vi "overlay_spot_circle.vi"(2 "Bubble Size":dbl, 4 "ID":dbl, 5 "error in":errorcluster, 6 "color(black)":u32, 7 "Position":cluster{"x":dbl, "y":dbl, "z":dbl}, 8 "image":T3) -> (0 "error out":errorcluster, 3 "Image Out":T3)   [LabVIEW 2019]
uses:
  <vilib>/vision/Image Controls.llb/IMAQ Image.ctl
  spot.ctl
  line_trapping.ctl
panel:
  in  "Spot Storage":T1[](array[typedef]) {"Amplitude Correction" step=0.1; "Line Trapping"."Phase Gradient" step=0.05; "Line Trapping"."Vector"."x" step=1e-06 format="%#_6p"; "Line Trapping"."Vector"."y" step=1e-06 format="%#_6p"; "Line Trapping"."Vector"."z" step=1e-06 format="%#_6p"; "NA Position"."r" step=1e-06; "NA Position"."y" step=1e-06; "NA Position"."x" step=1e-06; "Position"."z" step=1e-06; "Position"."y" step=1e-06; "Position"."x" step=1e-06; "Phase" step=0.7753; "Intensity" step=0.1}
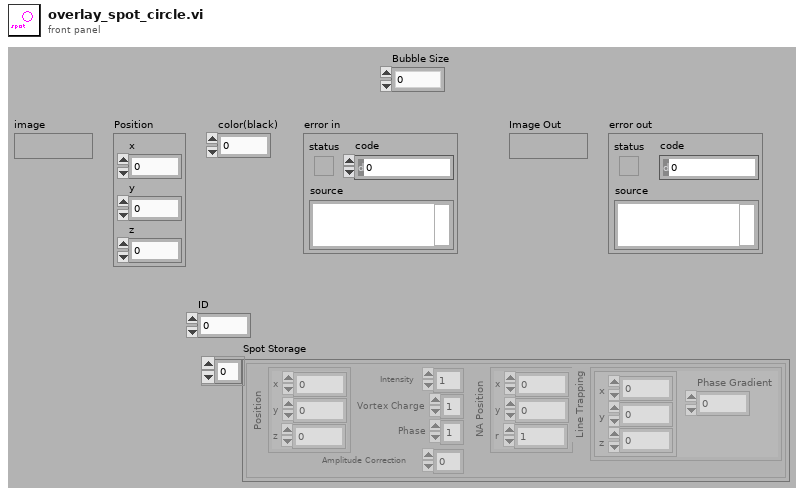
[diagram p1: front panel]
types:
  T1 = typedef "spot.ctl" = cluster{"Position":cluster{"x":dbl, "y":dbl, "z":dbl}, "Intensity":dbl, "Vortex Charge":i8, "Phase":dbl, "NA Position":cluster{"x":dbl, "y":dbl, "r":dbl}, "Line Trapping":T2, "Amplitude Correction":dbl}
  T2 = typedef "line_trapping.ctl" = cluster{"Vector":cluster{"x":dbl, "y":dbl, "z":dbl}, "Phase Gradient":dbl}
  T3 = typedef "IMAQ Image.ctl" = refnum<image>
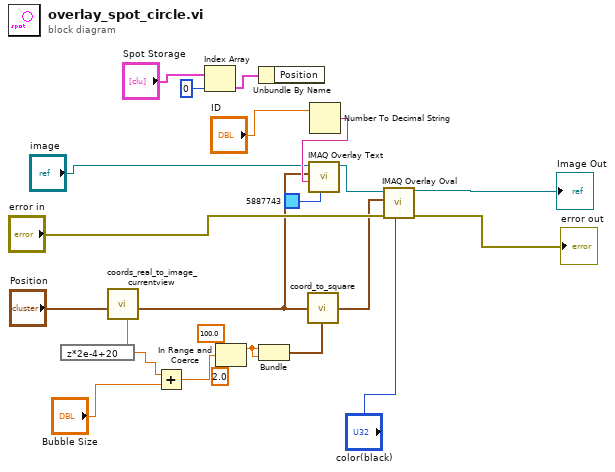
[diagram p0: block diagram]
diagram:
  n1 = call "coords_real_to_image_currentview.vi"("Position (real coords)"="Position") -> ("Position (pixels, relative to the top left of the image)"=w10:cluster{dbl, dbl}, "z (real coords)"=w19:dbl)  [unwired: 7 in]
  n2 = expression code="z*2e-4+20"(w19) -> (w3:dbl)
  n3 = Add(x=w3, y="Bubble Size") -> (x+y=w1:dbl)
  n4 = Index Array(array="Spot Storage", index=0) -> (element=w5:T1)
  n5 = In Range and Coerce(upper limit=100.0, x=w1, lower limit=2.0) -> (coerced(x)=w20:dbl)  [unwired: 1 out]
  n6 = Unbundle By Name(w5) -> ()  [unwired: 1 out]
  n7 = Bundle("upper limit"=w20, "upper limit"=w20) -> (w16:cluster{"upper limit":dbl, "upper limit":dbl})  [unwired: 1 in]
  n8 = call "coord_to_square.vi"("Size"=w16, "Centre"=w10) -> ("rectangle"=w21:cluster{dbl, dbl, dbl, dbl})  [unwired: 2 in]
  n9 = Number To Decimal String(number="ID") -> (decimal integer string=w12:string)  [unwired: 1 in]
  n10 = call "IMAQ Overlay Text"("Text Color (black)"=u32 5887743, "String"=w12, "Origin"=w10, "Image"="image") -> ("Image Out"=w9:T3)  [unwired: 6 in, 1 out]
  n11 = call "IMAQ Overlay Oval"("Color"="color(black)", "error in (no error)"="error in", "Bounding Rectangle"=w21, "Image"=w9) -> ("error out"=→"error out":errorcluster, "Image Out"=→"Image Out":T3)  [unwired: 6 in]
